vi "Log Assert Core.vi"(0 "Assert Name":string, 1 "Data Value":variant, 2 "Status":bool, 3 "Assert VI Name":string, 4 "Calling VI Name":string, 6 "Failure Action":T1, 7 "Assert Builder User Name":string, 8 "Last Update":timestamp, 9 "Assert Build Timestamp":timestamp, 10 "Evaluation String":string, 11 "Assert VI UID":i32, 12 "Comment":string, 13 "VI References":T2, 14 "Data Type":string) -> ()   [LabVIEW 2016, in "Assert API Components.lvlib"]
doc: "Core VI which logs all information for each assert and is scripted into each new assert vi.\nSet to Shared Clone Reentrant execution to prevent the assert API causing threadblocks within large applications."
uses:
  Assert API Components.lvlib
  VI References.ctl
  Failure Actions.ctl
  Message Data.ctl
  Log Assert Core Components/Log Assert Core.lvlib
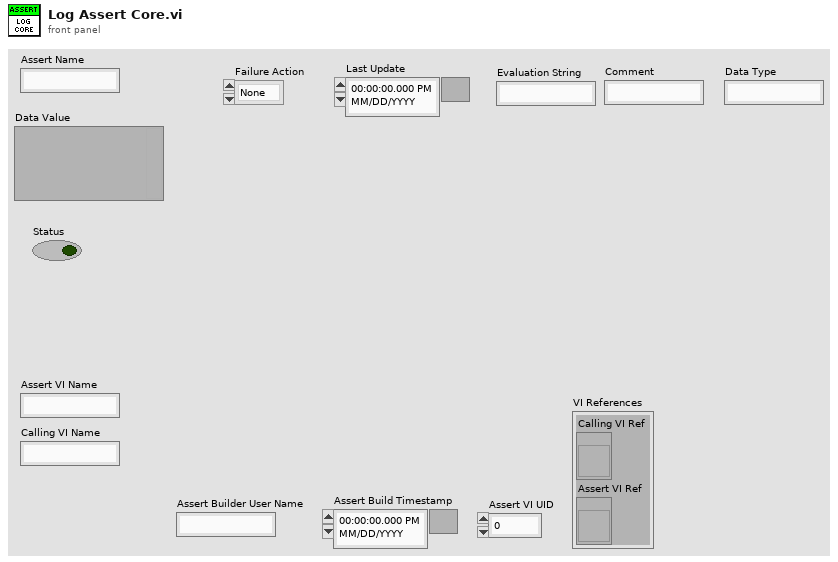
[diagram p1: front panel]
types:
  T1 = typedef "Assert API Components.lvlib/Failure Actions.ctl" = enum16{"None", "Log To File", "Pause Execution", "Abort Execution"}
  T2 = typedef "Assert API Components.lvlib/VI References.ctl" = cluster{"Calling VI Ref":refnum<vi>, "Assert VI Ref":refnum<vi>}
  T3 = typedef "Assert API Components.lvlib/Message Data.ctl" = cluster{"Data Value":variant, "Last Update":timestamp, "Comment":string, "Evaluation String":string, "Status":bool, "Assert Name":string, "Failure Action":T1, "Assert VI Name":string, "Calling VI Name":string, "Assert VI UID":i32, "Top Level VI Name":string, "VI References":T2, "Assert Build Timestamp":timestamp, "Assert Builder User Name":string, "Data Type":string, "IP Address":string}
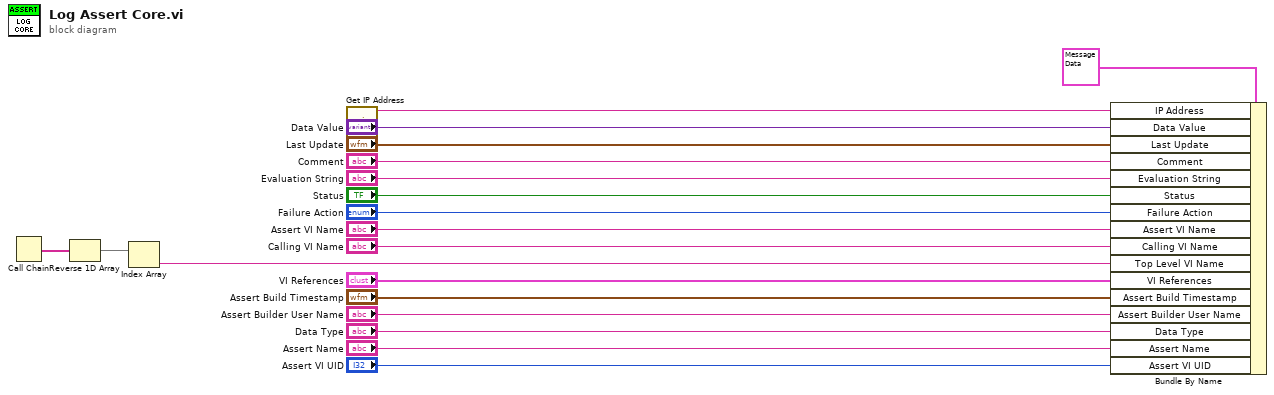
[diagram p0: block diagram]
diagram:
  n1 = Call Chain() -> (call chain=w5:string[])
  n2 = Reverse 1D Array(array=w5) -> (reversed array=w4:string[])
  n3 = Index Array(array=w4) -> (element=w3:string)  [unwired: 1 in]
  n4 = call "Get IP Address.vi"() -> ("IP Address"=w2:string)  [unwired: 11 in]
  n5 = Bundle By Name(cluster=T3 {"Data Value"=variant, "Last Update"=timestamp(0 s since 1904-01-01), "Comment"="", "Evaluation String"="", "Status"=FALSE, "Assert Name"="", "Failure Action"=enum."None", "Assert VI Name"="", "Calling VI Name"="", "Assert VI UID"=0, "Top Level VI Name"="", "VI References"={"Calling VI Ref"=refnum, "Assert VI Ref"=refnum}, "Assert Build Timestamp"=timestamp(0 s since 1904-01-01), "Assert Builder User Name"="", "Data Type"="", "IP Address"=""} ("Assert Message"), "IP Address"=w2, "Data Value"="Data Value", "Last Update"="Last Update", "Comment"="Comment", "Evaluation String"="Evaluation String", "Status"="Status", "Failure Action"="Failure Action", "Assert VI Name"="Assert VI Name", "Calling VI Name"="Calling VI Name", "Top Level VI Name"=w3, "VI References"="VI References", "Assert Build Timestamp"="Assert Build Timestamp", "Assert Builder User Name"="Assert Builder User Name", "Data Type"="Data Type", "Assert Name"="Assert Name", "Assert VI UID"="Assert VI UID") -> ()  [unwired: 1 out]
